vi "Target Main_copy.vi"() -> ()   [LabVIEW 2021]
uses:
  <vilib>/gmath/NumericalOptimization/stopping criteria.ctl
  <vilib>/Platform/TimedLoop/XDataNode/timing_clust.ctl
  <vilib>/Platform/TimedLoop/XDataNode/nitl_modes.ctl
  <vilib>/Platform/TimedLoop/XDataNode/wakeup.ctl
  <vilib>/Analysis/baseanly.llb/Real Dot Product.vi
  <vilib>/DAQmx/configure/timing.llb/DAQmx Timing (Sample Clock).vi
  <vilib>/DAQmx/miscellaneous.llb/DAQmx Fill In Error Info.vi
  <vilib>/platform/TimedLoop/XDataNode/XDataNode.xnode
  <vilib>/DAQmx/read.llb/DAQmx Read (Digital Bool 1Line 1Point).vi
  <vilib>/DAQmx/create/channels.llb/DAQmx Create Channel (AI-Voltage-Basic).vi
  <vilib>/DAQmx/create/channels.llb/DAQmx Create Channel (AO-Voltage-Basic).vi
  <vilib>/DAQmx/create/channels.llb/DAQmx Create Channel (DO-Digital Output).vi
  <vilib>/Analysis/Matrix/Numeric/Conversions/Matrix To Array - RM.vi
  <vilib>/DAQmx/write.llb/DAQmx Write (Analog 1D DBL NChan 1Samp).vi
  <vilib>/DAQmx/write.llb/DAQmx Write (Digital 1D Bool 1Chan 1Samp).vi
  <vilib>/DAQmx/create/channels.llb/DAQmx Create Channel (DI-Digital Input).vi
  <vilib>/Platform/TimedLoop/XDataNode/XDNodeRunTimeDep.lvlib
  <vilib>/Analysis/Matrix/NI_Matrix.lvlib
  <vilib>/Analysis/NI_AALBase.lvlib
  <vilib>/gmath/NI_Gmath.lvlib
panel:
  in  "threshold":dbl=0.05 format="%#_13g"
  in  "Learning Rate 2":dbl=0.0003 format="%#_13g"
  in  "Learning Rate":dbl=0.007 format="%#_13g"
  in  "Forgetting Factor":dbl=15.0 format="%#_13g"
  in  "Forgetting Factor":dbl=20.0 format="%#_13g"
  out "Reference Tension":dbl[](array[numeric])=[58.52912563704345, 70.0, 9.999999999999998]
  out "Cable Length":dbl[](array[numeric])=[1931.990998049138, 1130.3757457301724, 1657.5889594751345]
  in  "Resist Initialize":bool
  out "Record Start":bool
  in  "Assist Initialize":bool
  in  "Train":bool
  in  "Train?":bool
  out "Measured Phase":dbl=0.058742114867071954
  out "Reference Phase":dbl
  in  "Vitrual Spring":dbl(slide)=0.8 scale=0.0..1.0
  out "Trajectory Trigger":i32
  in  "default damp":dbl=0.001 format="%#_13g"
  in  "Learned Damping":bool
  out "Velocity Damping":dbl=0.02 format="%.2f"
  in  "Learned Stifffness":bool
  out "RBFN Virtual Spring":dbl=0.017398863416164045
  out "InRange Voltage":dbl[](array[slide]) scale=-5.0..5.0
  out "100ms Finished Late?":bool
  out "100ms":i64=20
  out "1ms Finished Late?":bool
  in  "Tension Control Gains":T1(array[cluster])=[{"proportional gain (Kc)"=0.1, "integral time (Ti, min)"=0.0, "derivative time (Td, min)"=0.0}, {"proportional gain (Kc)"=0.1, "integral time (Ti, min)"=0.0, "derivative time (Td, min)"=0.0}, {"proportional gain (Kc)"=0.1, "integral time (Ti, min)"=0.0, "derivative time (Td, min)"=0.0}] {"derivative time (Td, min)" format="%.3f"; "integral time (Ti, min)" format="%.3f"; "proportional gain (Kc)" format="%.3f"}
  out "1ms":i64=2
  out "10ms Finished Late?":bool
  out "10ms":i64=10
  in  "QP Stopping Criteria":T2={"function tolerance"=0.001, "parameter tolerance"=1e-05, "max iterations"=50, "max function calls"=50, "gradient tolerance"=1e-05, "max time (sec)"=0.01}
  in  "QP?":bool=TRUE
  out "QP Solved":bool=TRUE
  # "Manual"
  # "AAN"
  # "RAN"
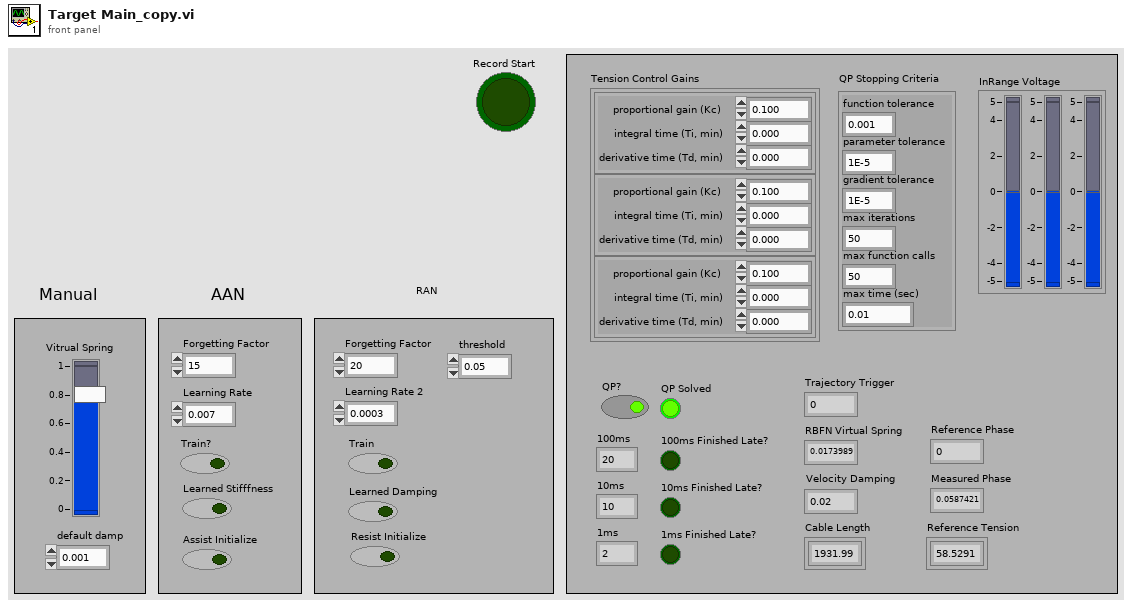
[diagram p1: front panel]
types:
  T1 = cluster{"proportional gain (Kc)":dbl, "integral time (Ti, min)":dbl, "derivative time (Td, min)":dbl}[]
  T2 = typedef "NI_Gmath.lvlib/stopping criteria.ctl" = cluster{"function tolerance":dbl, "parameter tolerance":dbl, "max iterations":i32, "max function calls":i32, "gradient tolerance":dbl, "max time (sec)":dbl}
  T3 = typedef "XDNodeRunTimeDep.lvlib/timing_clust.ctl" = cluster{"Expected End [f-1]":u64, "Actual End [f-1]":u64, "Finished Late? [f-1]":bool, "Expected End [i-1]":u64, "Actual End [i-1]":u64, "Finished Late? [i-1]":bool, "Expected Start [i]":u64, "Actual Start [i]":u64, "Expected Start [f]":u64, "Actual Start [f]":u64, "Source Name":string, "Structure Name":string, "Period":i64, "Deadline":i64, "Offset":i64, "Start":i64, "Priority":i32, "Timeout":i32, "Mode":T4, "Wakeup Reason":T5, "Error":errorcluster, "Source Type":string, "Secondary Source Type":string, "Global End Time":u64, "Global Start Time":u64, "Frame Duration":u64, "Iteration Duration":u64, "Assigned CPU":i32, "I/O Scan Engine Mode":u32}
  T4 = typedef "XDNodeRunTimeDep.lvlib/nitl_modes.ctl" = enum32{"No Change", "Process missed periods, maintain original phase", "Discard missed periods, maintain original phase", "Process missed periods, ignore original phase", "Discard missed periods, ignore original phase"}
  T5 = typedef "XDNodeRunTimeDep.lvlib/wakeup.ctl" = enum32{"Normal", "Aborted", "Asynchronous wakeup", "Timing source error", "Timed loop error", "Timeout"}
  T6 = typedef "NI_Matrix.lvlib/RealMatrix.ctl" = dbl[][]
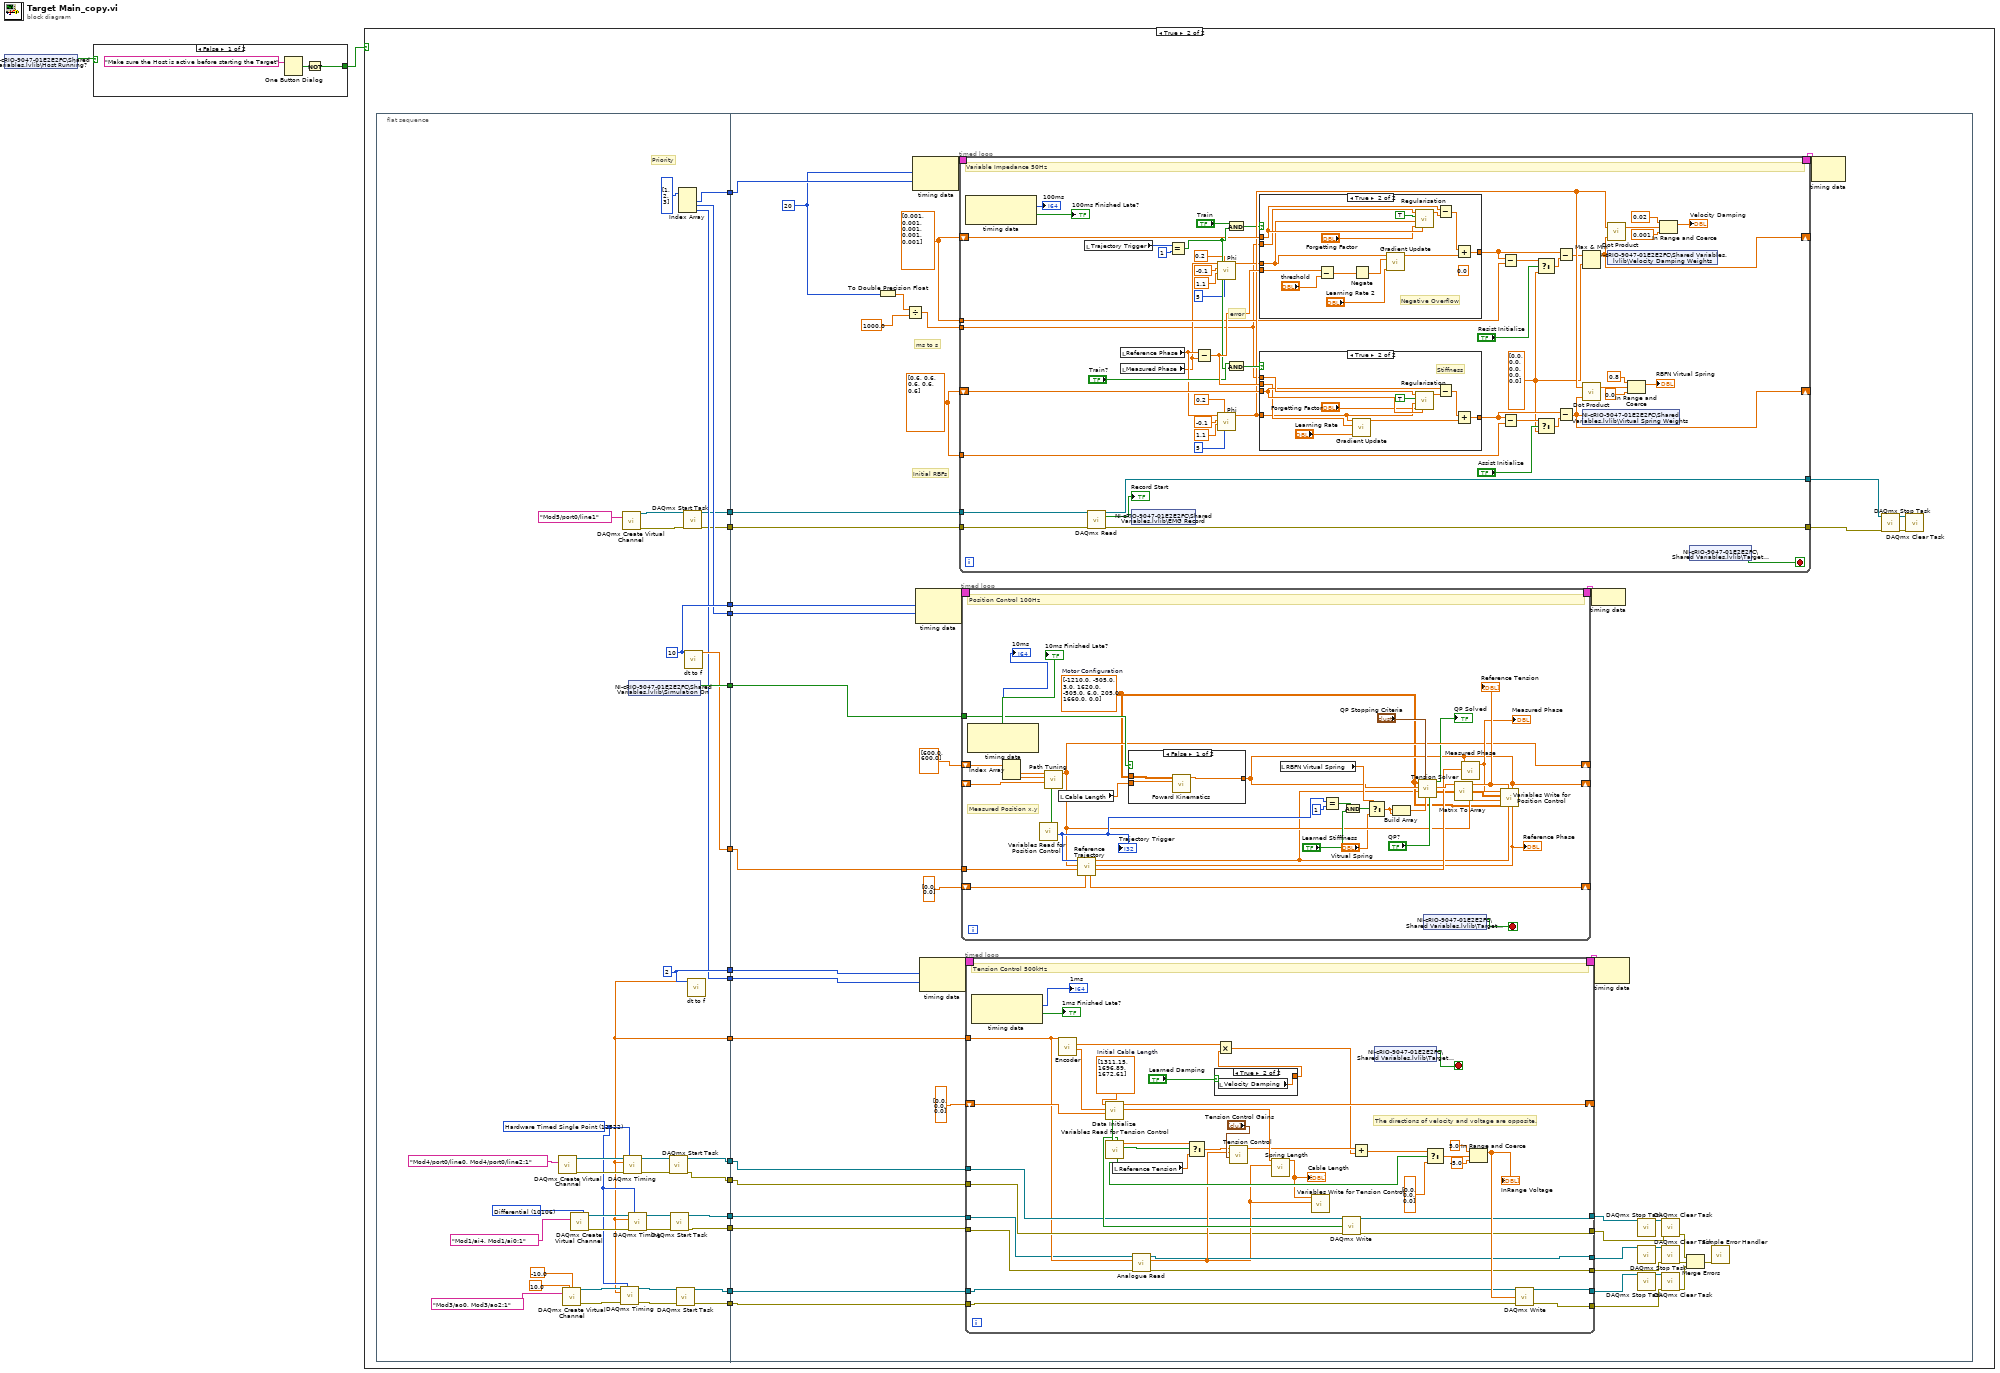
[diagram p0: block diagram]
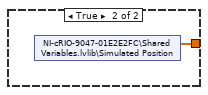
[diagram p5: hidden frame]
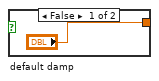
[diagram p6: hidden frame]
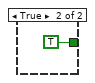
[diagram p7: hidden frame]
diagram:
  n1 = shared-variable "NI-cRIO-9047-01E2E2FC\\Shared Variables.lvlib\\Host Running?"() -> (w1:bool)  [unwired: 1 in, 1 out]
  n2 = case shown="False" w1 {
    tunnel: [w3 TRUE] -> w2
    frame False {
      n3 = One Button Dialog(message="Make sure the Host is active before starting the Target") -> (true=w4:bool)  [unwired: 1 in]
      n4 = Not(x=w4) -> (.not. x?=w3:bool)
    }
    frame True {
    }
  }
  n5 = case shown="True" w2 {
    frame False {
    }
    frame True {
      n6 = flat-sequence {
        tunnel: [w61] -> w22
        tunnel: [w60] -> w21
        tunnel: [w58] -> w20
        tunnel: [w57] -> w19
        tunnel: [w51] -> w18
        tunnel: [w28] -> w17
        tunnel: [w42] -> w16
        tunnel: [w41] -> w15
        tunnel: [w40] -> w14
        tunnel: [w39] -> w13
        tunnel: [w38] -> w12
        tunnel: [w36] -> w11
        tunnel: [w35] -> w10
        tunnel: [w34] -> w9
        tunnel: [w27] -> w8
        tunnel: [w26] -> w7
        tunnel: w22 -> [w90]
        tunnel: w21 -> [w89]
        tunnel: w20 -> [w87]
        tunnel: w19 -> [w86]
        tunnel: w18 -> [w85]
        tunnel: w17 -> [w84]
        tunnel: w16 -> [w83]
        tunnel: w15 -> [w82]
        tunnel: w14 -> [w81]
        tunnel: w13 -> [w80]
        tunnel: w12 -> [w78]
        tunnel: w11 -> [w77]
        tunnel: w10 -> [w79]
        tunnel: w9 -> [w88]
        tunnel: w8 -> [w69]
        tunnel: w7 -> [w68]
        frame #0 {
          w29 = 12522 items=["Finite Samples"=10178, "Continuous Samples"=10123, "Hardware Timed Single Point"=12522] ("sample mode")
          w50 = 10106 items=["Default"=-1, "RSE"=10083, "NRSE"=10078, "Differential"=10106, "Pseudodifferential"=12529] ("input terminal configuration")
          w51 = i64 2 ("Period")
          w60 = i64 10 ("Period 3")
          # "Priority"
          n7 = call-poly <vilib>:"DAQmx Create Virtual Channel.vi"("lines"=tag "Mod4/port0/line0, Mod4/port0/line2:1") -> ("task out"=w33:refnum<k21>, "error out"=w30:errorcluster)  [unwired: 13 in]
          n8 = call-poly <vilib>:"DAQmx Create Virtual Channel.vi"("maximum value"=10.0 ("AO max"), "minimum value"=-10.0 ("AO min"), "physical channels"=tag "Mod3/ao0, Mod3/ao2:1" ("Physical Channel(s)")) -> ("task out"=w53:refnum<k21>, "error out"=w52:errorcluster)  [unwired: 11 in]
          n9 = call-poly <vilib>:"DAQmx Create Virtual Channel.vi"("input terminal configuration"=w50, "physical channels"=tag "Mod1/ai4, Mod1/ai0:1") -> ("task out"=w48:refnum<k21>, "error out"=w47:errorcluster)  [unwired: 12 in]
          n10 = call-poly <vilib>:"DAQmx Create Virtual Channel.vi"("lines"=tag "Mod5/port0/line1") -> ("task out"=w24:refnum<k21>, "error out"=w23:errorcluster)  [unwired: 13 in]
          n11 = shared-variable "NI-cRIO-9047-01E2E2FC\\Shared Variables.lvlib\\Simulation On"() -> (w61:bool)  [unwired: 1 in, 1 out]
          n12 = Index Array(array=i32[] [1, 2, 3]) -> (element #1=w36:i32, element #2=w34:i32, element #3=w35:i32)  [unwired: 3 in]
          n13 = call <vilib>:"DAQmx Start Task.vi"("task/channels in"=w24, "error in"=w23) -> ("task out"=w27:refnum<k21>, "error out"=w26:errorcluster)  [unwired: 12 in]
          n14 = call "dt to f.vi"("Period"=w60) -> ("Frequency"=w38:dbl)  [unwired: 10 in]
          n15 = call "dt to f.vi"("Period"=w51) -> ("Frequency"=w28:dbl)  [unwired: 10 in]
          n16 = call-poly <vilib>:"DAQmx Timing.vi"("task/channels in"=w53, "sample mode"=w29, "rate"=w28, "error in"=w52) -> ("task out"=w44:refnum<k21>, "error out"=w43:errorcluster)  [unwired: 10 in]
          n17 = call-poly <vilib>:"DAQmx Timing.vi"("task/channels in"=w33, "sample mode"=w29, "rate"=w28, "error in"=w30) -> ("task out"=w32:refnum<k21>, "error out"=w31:errorcluster)  [unwired: 10 in]
          n18 = call-poly <vilib>:"DAQmx Timing.vi"("task/channels in"=w48, "sample mode"=w29, "rate"=w28, "error in"=w47) -> ("task out"=w46:refnum<k21>, "error out"=w45:errorcluster)  [unwired: 10 in]
          n19 = call <vilib>:"DAQmx Start Task.vi"("task/channels in"=w32, "error in"=w31) -> ("task out"=w58:refnum<k21>, "error out"=w57:errorcluster)  [unwired: 12 in]
          n20 = call <vilib>:"DAQmx Start Task.vi"("task/channels in"=w46, "error in"=w45) -> ("task out"=w42:refnum<k21>, "error out"=w41:errorcluster)  [unwired: 12 in]
          n21 = call <vilib>:"DAQmx Start Task.vi"("task/channels in"=w44, "error in"=w43) -> ("task out"=w40:refnum<k21>, "error out"=w39:errorcluster)  [unwired: 12 in]
        }
        frame #1 {
          w63 = dbl[] [0.6, 0.6, 0.6, 0.6, 0.6] ("Array of Double")
          w62 = dbl[] [0.001, 0.001, 0.001, 0.001, 0.001]
          w72 = i64 20 ("Period 3")
          # "Initial RBFs"
          # "ms to s"
          n22 = To Double Precision Float(number=w72) -> (double precision float=w71:dbl)
          n23 = Divide(x=w71, y=1000.0) -> (x/y=w70:dbl)
          n24 = node-c288(w72, w77) -> (w105:T3)
          n25 = node-c288(w89, w88) -> (w107:T3)
          n26 = node-c288(w85, w79) -> (w109:T3)
          n27 = timed-loop {
            timing: w105 -> [_]
            timing-out: [_] -> w104
            tunnel: w70 -> [w110]
            shift-right: [w127] -> _
            shift-left: w63 -> [w155]
            shift-right: [w111] -> _
            shift-left: w62 -> [w144]
            tunnel: w69 -> [w141]
            tunnel: w68 -> [w140]
            tunnel: [w138] -> w66
            tunnel: [w139] -> w64
            tunnel: w63 -> [w122]
            tunnel: w62 -> [w121]
            stop <- w160 stop-if-true
            w112 = dbl[] [0.0, 0.0, 0.0, 0.0, 0.0] ("Array of Double")
            # "error"
            # "Variable Impedance 50Hz"
            n28 = node-c288() -> (→"100ms":i64, →"100ms Finished Late?":bool)  [unwired: 1 in]
            n29 = local read "Trajectory Trigger"() -> (w148:i32)
            n30 = call-poly <vilib>:"DAQmx Read.vi"("task/channels in"=w141, "error in"=w140) -> ("task out"=w138:refnum<k21>, "data"=w137:bool, "error out"=w139:errorcluster)  [unwired: 11 in]
            "Record Start" <- w137
            n31 = local read "Reference Phase"() -> (w120:dbl)
            n32 = local read "Measured Phase"() -> (w118:dbl)
            n33 = shared-variable "NI-cRIO-9047-01E2E2FC\\Shared Variables.lvlib\\EMG Record"(w137) -> ()  [unwired: 1 in, 1 out]
            n34 = Equal?(x=w148, y=1) -> (x = y?=w145:bool)
            n35 = Subtract(x=w120, y=w118) -> (x-y=w150:dbl)
            n36 = call "Phi.vi"("Number"=5, "STD"=0.2 ("x_0"), "x_f"=1.1, "x_0"=-0.1, "X (mm)"=w118) -> ("Phi"=w119:dbl[])  [unwired: 6 in]
            n37 = call "Phi.vi"("Number"=5, "STD"=0.2, "x_f"=1.1, "x_0"=-0.1, "X (mm)"=w120) -> ("Phi"=w142:dbl[])  [unwired: 6 in]
            n38 = And(x="Train", y=w145) -> (x .and. y?=w131:bool)
            n39 = And(x="Train?", y=w145) -> (x .and. y?=w146:bool)
            n40 = case shown="True" w131 {
              tunnel: w150 -> [_ w173]
              tunnel: w119 -> [_ w175]
              tunnel: w144 -> [w163 w177]
              tunnel: [w163 w176] -> w124
              tunnel: w110 -> [_ w171]
              frame False {
              }
              frame True {
                (unwired) 0.0 ("t")
                # "Negative Overflow"
                n41 = Subtract(x=w173, y="threshold") -> (x-y=w172:dbl)
                n42 = Negate(x=w172) -> (-x=w169:dbl)
                n43 = call "Gradient Update.vi"("Learning Rate"="Learning Rate 2", "Error"=w169, "Phi"=w175) -> ("Gradient Update"=w170:dbl[])  [unwired: 8 in]
                n44 = call "Regularisation.vi"("W"=w177, "tau_f"="Forgetting Factor", "Phi"=w175, "Forgetting?"=TRUE, "dt"=w171) -> ("Forgetting Term"=w167:dbl[])  [unwired: 6 in]
                n45 = Subtract(x=w177, y=w167) -> (x-y=w165:dbl[])
                n46 = Add(x=w165, y=w170) -> (x+y=w176:dbl[])
              }
            }
            n47 = case shown="True" w146 {
              tunnel: w110 -> [_ w189]
              tunnel: w155 -> [w178 w188]
              tunnel: w142 -> [_ w185]
              tunnel: w150 -> [_ w186]
              tunnel: [w178 w182] -> w126
              frame False {
              }
              frame True {
                # "Stiffness"
                n48 = call "Gradient Update.vi"("Learning Rate"="Learning Rate", "Error"=w186, "Phi"=w185) -> ("Gradient Update"=w184:dbl[])  [unwired: 8 in]
                n49 = call "Regularisation.vi"("W"=w188, "tau_f"="Forgetting Factor", "Phi"=w185, "Forgetting?"=TRUE, "dt"=w189) -> ("Forgetting Term"=w187:dbl[])  [unwired: 6 in]
                n50 = Subtract(x=w188, y=w187) -> (x-y=w183:dbl[])
                n51 = Add(x=w183, y=w184) -> (x+y=w182:dbl[])
              }
            }
            n52 = Subtract(x=w124, y=w121) -> (x-y=w123:dbl[])
            n53 = Subtract(x=w126, y=w122) -> (x-y=w125:dbl[])
            n54 = Select(t=w123, s="Resist Initialize", f=w112) -> (s? t:f=w128:dbl[])
            n55 = Select(t=w125, s="Assist Initialize", f=w112) -> (s? t:f=w136:dbl[])
            n56 = Subtract(x=w124, y=w128) -> (x-y=w113:dbl[])
            n57 = Subtract(x=w126, y=w136) -> (x-y=w127:dbl[])
            n58 = Max & Min(x=w113, y=w112) -> (max(x,y)=w111:dbl[])  [unwired: 1 out]
            n59 = call-poly <vilib>:"Dot Product.vi"("Y Vector"=w127, "X Vector"=w142) -> ("X * Y"=w152:dbl)  [unwired: 1 out]
            n60 = shared-variable "NI-cRIO-9047-01E2E2FC\\Shared Variables.lvlib\\Virtual Spring Weights"(w127) -> ()  [unwired: 1 in, 1 out]
            n61 = call-poly <vilib>:"Dot Product.vi"("Y Vector"=w111, "X Vector"=w142) -> ("X * Y"=w130:dbl)  [unwired: 1 out]
            n62 = shared-variable "NI-cRIO-9047-01E2E2FC\\Shared Variables.lvlib\\Velocity Damping Weights"(w111) -> ()  [unwired: 1 in, 1 out]
            n63 = In Range and Coerce(upper limit=0.8, x=w152, lower limit=0.0) -> (coerced(x)=→"RBFN Virtual Spring":dbl)  [unwired: 1 out]
            n64 = In Range and Coerce(upper limit=0.02, x=w130, lower limit=0.001) -> (coerced(x)=→"Velocity Damping":dbl)  [unwired: 1 out]
            n65 = shared-variable "NI-cRIO-9047-01E2E2FC\\Shared Variables.lvlib\\Target Stop"() -> (w160:bool)  [unwired: 1 in, 1 out]
          }
          n66 = timed-loop {
            timing: w107 -> [_]
            timing-out: [_] -> w106
            tunnel: w90 -> [w226]
            shift-right: [w203] -> _
            shift-left: _ -> [w214]
            tunnel: w78 -> [w213]
            shift-right: [w211] -> _
            shift-left: dbl[] [600.0, 600.0] -> [w212]
            shift-right: [w209] -> _
            shift-left: dbl[] [0.0, 0.0] -> [w210]
            stop <- w225 stop-if-true
            w202 = dbl[][] [[-1210.0, -505.0, 3.0], [1620.0, -505.0, 6.0], [205.0, 1660.0, 0.0]]  # Motor Configuration
            # "Measured Position x,y"
            # "Position Control 100Hz"
            n67 = node-c288() -> (→"10ms":i64, →"10ms Finished Late?":bool)  [unwired: 1 in]
            n68 = Index Array(array=w212) -> (element #1=w207:dbl, element #2=w206:dbl)  [unwired: 2 in]
            n69 = call "Variables Read for Position Control.vi"() -> ("Trajectory Trigger"=w224:i32, "Start, End Point"=w205:bool[])  [unwired: 10 in]
            "Trajectory Trigger" <- w224
            n70 = call "Path Tuning.vi"("Tune"=w205, "Measured Position"=w214, "Default Y"=w206, "Default X"=w207) -> ("Ellipse Length"=w211:dbl[])  [unwired: 7 in]
            n71 = local read "Cable Length"() -> (w200:dbl[])
            n72 = call "Reference Trajectory.vi"("Trajectory Time in"=w210, "Frequency"=w213, "Ellipse Length"=w211, "Trajectory Trigger"=w224) -> ("Total Phase"=w227:dbl, "Reference Phase"=w208:dbl, "Reference X,Y"=w199:dbl[], "Trajectory Time out"=w209:dbl[])  [unwired: 4 in]
            "Reference Phase" <- w208
            n73 = case shown="False" w226 {
              tunnel: [w239 w240] -> w203
              tunnel: w202 -> [w238 _]
              tunnel: w200 -> [w237 _]
              frame False {
                n74 = call "Foward Kinematics.vi"("Cable Length"=w237, "Motor Configuration"=w238) -> ("Measured Position"=w239:dbl[])  [unwired: 9 in]
              }
              frame True {
                n75 = shared-variable "NI-cRIO-9047-01E2E2FC\\Shared Variables.lvlib\\Simulated Position"() -> (w240:dbl[])  [unwired: 1 in, 1 out]
              }
            }
            n76 = local read "RBFN Virtual Spring"() -> (w222:dbl)
            n77 = Equal?(x=w224, y=1) -> (x = y?=w217:bool)
            n78 = And(x=w217, y="Learned Stifffness") -> (x .and. y?=w216:bool)
            n79 = Select(t=w222, s=w216, f="Vitrual Spring") -> (s? t:f=w221:dbl)
            n80 = Build Array(w221, w221) -> (w220:dbl[])
            n81 = call "Tension Solver.vi"("QP?"="QP?", "P Gain"=w220, "QP Stopping Criteria"="QP Stopping Criteria", "Reference X,Y"=w199, "Measured Position"=w203, "Motor Configuration"=w202) -> ("Jacobian"=w219:T6, "Reference Tension"=w229:dbl[], "QP Solved"=→"QP Solved":bool)  [unwired: 3 in]
            "Reference Tension" <- w229
            n82 = shared-variable "NI-cRIO-9047-01E2E2FC\\Shared Variables.lvlib\\Target Stop"() -> (w225:bool)  [unwired: 1 in, 1 out]
            n83 = call-poly <vilib>:"Matrix To Array.vi"("Real Matrix"=w219) -> ("Real 2D Array"=w218:dbl[][])
            n84 = call "Measured Phase.vi"("Total Phase"=w227, "Measured Position"=w203) -> ("Measured Phase"=w228:dbl)  [unwired: 9 in]
            "Measured Phase" <- w228
            n85 = call "Variables Write for Position Control.vi"("Reference Phase"=w208, "Measured Position"=w203, "Reference Position"=w199, "Reference Tension"=w229, "Motors Configuration"=w202, "Ellipse Length"=w211, "Jacobian"=w218, "Measured Phase"=w228) -> ()  [unwired: 4 in]
          }
          n86 = timed-loop {
            tunnel: [w269] -> w94
            tunnel: [w268] -> w97
            tunnel: [w271] -> w96
            tunnel: [w270] -> w98
            tunnel: [w273] -> w92
            shift-right: [w265] -> _
            shift-left: dbl[] [0.0, 0.0, 0.0] ("Encoder Position (mm)") -> [w263]
            timing: w109 -> [_]
            timing-out: [_] -> w108
            tunnel: [w272] -> w99
            tunnel: w87 -> [w258]
            tunnel: w86 -> [w257]
            tunnel: w84 -> [w256]
            tunnel: w83 -> [w255]
            tunnel: w82 -> [w254]
            tunnel: w81 -> [w253]
            tunnel: w80 -> [w252]
            stop <- w262 stop-if-true
            w266 = dbl[] [1311.15, 1696.89, 1672.61]  # Initial Cable Length
            # "The directions of velocity and voltage are opposite."
            # "Tension Control 500kHz"
            n87 = node-c288() -> (→"1ms":i64, →"1ms Finished Late?":bool)  [unwired: 1 in]
            n88 = call "Encoder.vi"("Frequency"=w256) -> ("Encoder Position (mm)"=w264:dbl[], "RPM"=w277:dbl[])  [unwired: 9 in]
            n89 = call "Variables Read for Tension Control.vi"() -> ("Manual Control?"=w275:bool, "Manual Control"=w274:dbl[], "Tension Control On"=w278:bool, "Motor Enable"=w283:bool[], "Encoder Initialize"=w284:bool)  [unwired: 7 in]
            n90 = call "Data Initialize.vi"("Initialize"=w284, "Compensation in"=w263, "Data in"=w264, "Set Data"=w266) -> ("Data out"=w261:dbl[], "Compensation out"=w265:dbl[])  [unwired: 6 in]
            n91 = local read "Reference Tension"() -> (w246:dbl[])
            n92 = call "Analogue Read.vi"("error in"=w254, "sampling freq: fs"=w256, "task/channels in"=w255) -> ("error out"=w270:errorcluster, "Measured Tension"=w259:dbl[], "task out"=w271:refnum<k21>)  [unwired: 6 in]
            n93 = Select(t=w274, s=w275, f=w246) -> (s? t:f=w276:dbl[])
            n94 = case shown="True" "Learned Damping" {
              tunnel: ["default damp" w289] -> w248
              frame False {
              }
              frame True {
                n95 = local read "Velocity Damping"() -> (w289:dbl)
              }
            }
            n96 = Multiply(x=w277, y=w248) -> (x*y=w250:dbl[])
            n97 = call "Tension Control.vi"("PID gains"="Tension Control Gains", "Measured Tension"=w259, "Reference Tension"=w276) -> ("Voltage Output"=w251:dbl[])  [unwired: 8 in]
            n98 = call "Spring Length.vi"("Measured Tension"=w259, "Cable Length in"=w261) -> ("Cable Length out"=w260:dbl[])  [unwired: 9 in]
            "Cable Length" <- w260
            n99 = call "Variables Write for Tension Control.vi"("Measured Tension"=w259, "Cable Length in"=w260) -> ()  [unwired: 10 in]
            n100 = call-poly <vilib>:"DAQmx Write.vi"("task/channels in"=w258, "data"=w283, "error in"=w257) -> ("task out"=w273:refnum<k21>, "error out"=w272:errorcluster)  [unwired: 10 in, 1 out]
            n101 = Add(x=w251, y=w250) -> (x+y=w249:dbl[])
            n102 = shared-variable "NI-cRIO-9047-01E2E2FC\\Shared Variables.lvlib\\Target Stop"() -> (w262:bool)  [unwired: 1 in, 1 out]
            n103 = Select(t=w249, s=w278, f=dbl[] [0.0, 0.0, 0.0]) -> (s? t:f=w285:dbl[])
            n104 = In Range and Coerce(upper limit=5.0, x=w285, lower limit=-5.0) -> (coerced(x)=w282:dbl[])  [unwired: 1 out]
            "InRange Voltage" <- w282
            n105 = call-poly <vilib>:"DAQmx Write.vi"("task/channels in"=w253, "data"=w282, "error in"=w252) -> ("task out"=w269:refnum<k21>, "error out"=w268:errorcluster)  [unwired: 10 in, 1 out]
          }
          n106 = node-c288(w106) -> ()
          n107 = node-c288(w108) -> ()  [unwired: 1 out]
          n108 = call <vilib>:"DAQmx Stop Task.vi"("task/channels in"=w92) -> ("task out"=w91:refnum<k21>)  [unwired: 13 in, 1 out]
          n109 = call <vilib>:"DAQmx Stop Task.vi"("task/channels in"=w96) -> ("task out"=w95:refnum<k21>)  [unwired: 13 in, 1 out]
          n110 = call <vilib>:"DAQmx Stop Task.vi"("task/channels in"=w94) -> ("task out"=w93:refnum<k21>)  [unwired: 13 in, 1 out]
          n111 = call <vilib>:"DAQmx Clear Task.vi"("task in"=w91, "error in"=w99) -> ("error out"=w103:errorcluster)  [unwired: 13 in]
          n112 = call <vilib>:"DAQmx Clear Task.vi"("task in"=w95, "error in"=w98) -> ("error out"=w102:errorcluster)  [unwired: 13 in]
          n113 = call <vilib>:"DAQmx Clear Task.vi"("task in"=w93, "error in"=w97) -> ("error out"=w101:errorcluster)  [unwired: 13 in]
          n114 = Merge Errors(w103, w102, w101) -> (w100:errorcluster)
          n115 = call <vilib>:"Simple Error Handler.vi"("error in (no error)"=w100) -> ()  [unwired: 4 in, 5 out]
          n116 = node-c288(w104) -> ()  [unwired: 1 out]
          n117 = call <vilib>:"DAQmx Stop Task.vi"("task/channels in"=w66, "error in"=w64) -> ("task out"=w67:refnum<k21>, "error out"=w65:errorcluster)  [unwired: 12 in]
          n118 = call <vilib>:"DAQmx Clear Task.vi"("task in"=w67, "error in"=w65) -> ()  [unwired: 13 in, 1 out]
        }
      }
    }
  }
